vi "Shutdown Progress Indicator.vi"(8 "error in":errorcluster) -> (0 "error out":errorcluster)   [LabVIEW 2013, in "LVTM.lvlib"]
uses:
  LVTM.lvlib
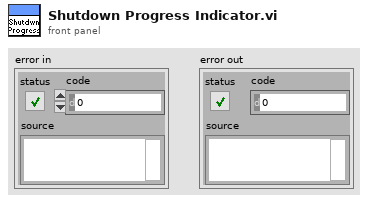
[diagram p1: front panel]
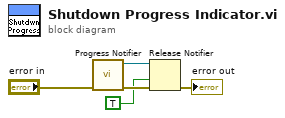
[diagram p0: block diagram]
diagram:
  n1 = call "Progress Notifier.vi"("error in"="error in") -> ("error out"=w3:errorcluster, "notifier out"=w2:refnum<notifier>)  [unwired: 9 in]
  n2 = Release Notifier(notifier=w2, force destroy? (F)=TRUE, error in (no error)=w3) -> (error out=→"error out":errorcluster)  [unwired: 2 out]
